vi "Introspection Core.vi"(8 "error in (no error)":errorcluster, 11 "CS++Scope in":refnum<class "CS++Scope.lvclass">) -> (0 "error out":errorcluster, 2 "CS++Messages":refnum<class "Message.lvclass">[](array[class]), 3 "CS++Scope out":refnum<class "CS++Scope.lvclass">)   [LabVIEW 2015, in "CS++Scope.lvlib" / "CS++Scope.lvclass"]
doc: "This vi delivers a list with all messages this actor reacts to. \n\nNote that all inherited classes have to overwrite it."
uses:
  CS++Scope.lvclass
  <vilib>/ActorFramework/Message/Message.lvclass
  CS++Scope Messages/Abort Msg/Abort Msg.lvclass
  CS++Scope Messages/Auto Setup Msg/Auto Setup Msg.lvclass
  CS++Scope Messages/Configure Acquisition Record Msg/Configure Acquisition Record Msg.lvclass
  CS++Scope Messages/Configure Acquisition Type Msg/Configure Acquisition Type Msg.lvclass
  CS++Scope Messages/Configure Channel Characteristics Msg/Configure Channel Characteristics Msg.lvclass
  CS++Scope Messages/Configure Channel Msg/Configure Channel Msg.lvclass
  CS++Scope Messages/Configure Edge Trigger Source Msg/Configure Edge Trigger Source Msg.lvclass
  CS++Scope Messages/Configure Trigger Coupling Msg/Configure Trigger Coupling Msg.lvclass
  CS++Scope Messages/Configure Trigger Msg/Configure Trigger Msg.lvclass
  CS++Scope Messages/Fetch Waveform Msg/Fetch Waveform Msg.lvclass
  CS++Scope Messages/Initiate Acquisition Msg/Initiate Acquisition Msg.lvclass
  CSPP_Core/Actors/CS++DeviceActor/CS++DeviceActor.lvclass
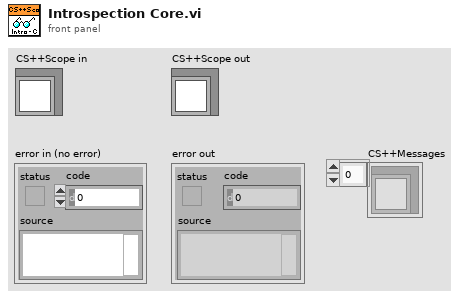
[diagram p1: front panel]
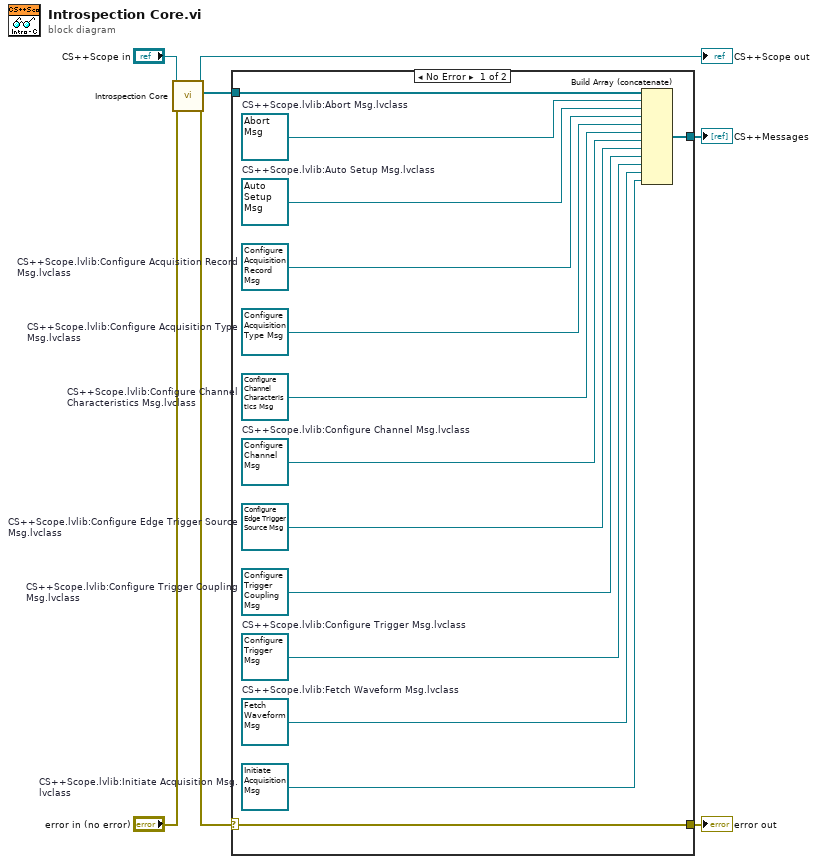
[diagram p0: block diagram]
diagram:
  n1 = call-parent "Introspection Core.vi"("error in (no error)"="error in (no error)", "CS++DeviceActor in"="CS++Scope in") -> ("error out"=w4:errorcluster, "CS++Messages"=w2:refnum<class "Message.lvclass">[], "CS++DeviceActor out"=→"CS++Scope out":refnum<class "CS++Scope.lvclass">)  [unwired: 7 in]
  n2 = case shown="No Error" w4 {
    selector: w4 -> [w21 w22]
    tunnel: [w21 w22] -> w3
    tunnel: w2 -> [w20 _]
    tunnel: [w8 _] -> w1
    frame No Error {
      w9 = refnum<class "Initiate Acquisition Msg.lvclass"> refnum  # CS++Scope.lvlib:Initiate Acquisition Msg.lvclass
      w10 = refnum<class "Fetch Waveform Msg.lvclass"> refnum  # CS++Scope.lvlib:Fetch Waveform Msg.lvclass
      w11 = refnum<class "Configure Trigger Msg.lvclass"> refnum  # CS++Scope.lvlib:Configure Trigger Msg.lvclass
      w12 = refnum<class "Configure Trigger Coupling Msg.lvclass"> refnum  # CS++Scope.lvlib:Configure Trigger Coupling Msg.lvclass
      w13 = refnum<class "Configure Edge Trigger Source Msg.lvclass"> refnum  # CS++Scope.lvlib:Configure Edge Trigger Source Msg.lvclass
      w14 = refnum<class "Configure Channel Msg.lvclass"> refnum  # CS++Scope.lvlib:Configure Channel Msg.lvclass
      w15 = refnum<class "Configure Channel Characteristics Msg.lvclass"> refnum  # CS++Scope.lvlib:Configure Channel Characteristics Msg.lvclass
      w16 = refnum<class "Configure Acquisition Type Msg.lvclass"> refnum  # CS++Scope.lvlib:Configure Acquisition Type Msg.lvclass
      w17 = refnum<class "Configure Acquisition Record Msg.lvclass"> refnum  # CS++Scope.lvlib:Configure Acquisition Record Msg.lvclass
      w18 = refnum<class "Auto Setup Msg.lvclass"> refnum  # CS++Scope.lvlib:Auto Setup Msg.lvclass
      w19 = refnum<class "Abort Msg.lvclass"> refnum  # CS++Scope.lvlib:Abort Msg.lvclass
      n3 = Build Array (concatenate)(w20, w19, w18, w17, w16, w15, w14, w13, w12, w11, w10, w9) -> (w8:refnum<class "Message.lvclass">[])
    }
    frame Error {
    }
  }
  "error out" <- w3
  "CS++Messages" <- w1
